vi "Set Symbol.vi"(7 "Skip If Worse (T)":bool=TRUE, 8 "error in (no error)":errorcluster, 9 "Test Outcome":T1, 10 "Tag Name":string, 11 "ResultTree in":refnum<class "ResultTree.lvclass">) -> (0 "error out":errorcluster, 3 "ResultTree out":refnum<class "ResultTree.lvclass">)   [LabVIEW 2017, in "ResultTree.lvclass"]
doc: "Sets the symbol for the specified tag name based on the provided test outcome. The default behavior is to skip tags whose outcome is already worse than the provided outcome."
uses:
  ResultTree.lvclass
  Test Outcome.ctl
  ResultTree.lvclass/ResultTree.ctl
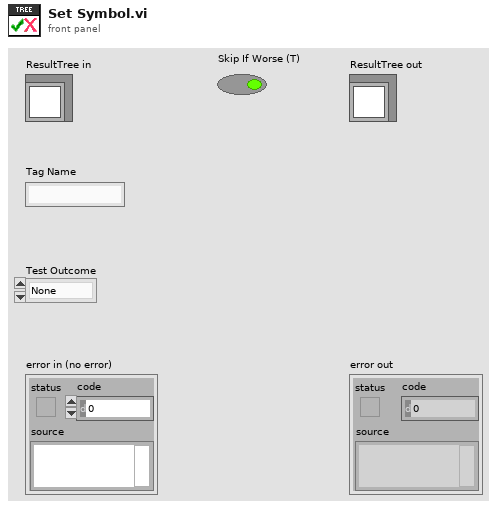
[diagram p1: front panel]
types:
  T1 = typedef "Test Outcome.ctl" = enum16{"None", "Passed", "Failed"}
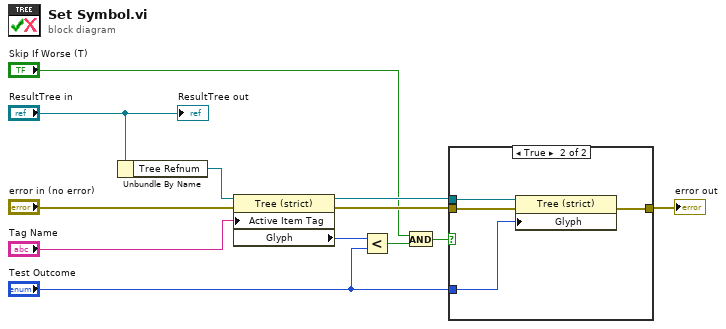
[diagram p0: block diagram]
diagram:
  n1 = Unbundle By Name("ResultTree in") -> ("Tree Refnum"=w10:refnum<vi>)
  n2 = property class="Tree (strict)"(reference=w10, error in="error in (no error)", "Active Item Tag"="Tag Name") -> (reference out=w6:refnum<vi>, error out=w8:errorcluster, "Glyph"=w4:i32)
  n3 = Less?(x=w4, y="Test Outcome") -> (x < y?=w5:bool)
  n4 = And(x="Skip If Worse (T)", y=w5) -> (x .and. y?=w2:bool)
  n5 = case shown="True" w2 {
    tunnel: [w13 w17] -> w12
    tunnel: "Test Outcome" -> [_ w16]
    tunnel: w8 -> [w13 w15]
    tunnel: w6 -> [_ w14]
    frame False {
    }
    frame True {
      n6 = property class="Tree (strict)"(reference=w14, error in=w15, "Glyph"=w16) -> (error out=w17:errorcluster)  [unwired: 1 out]
    }
  }
  "error out" <- w12
  "ResultTree out" <- "ResultTree in"
